vi "navX reading VI.vi"(0 "NavX Info In":T6, 1 "Mode":T7, 2 "error in (no error)":errorcluster) -> (3 "NavX Info Out":T6, 4 "NavX Readings":T4, 5 "Status":T3 {"OP Status" items=["INITIALIZING", "SELFTEST_IN_PROGRESS", "ERROR", "IMU_AUTOCAL_IN_PROGRESS", "NORMAL"]; "Calibration Status" items=["IMU_CAL_STATE_MASK"=3, "IMU_CAL_STATE_INPROGRESS"=0, "IMU_CAL_STATE_ACCUMULATE"=1, "IMU_CAL_STATE_COMPLETE"=2]}, 6 "Error Out":errorcluster)   [LabVIEW 2018]
uses:
  navX type def.ctl
  <vilib>/Studica/Studica Toolkit/Background/I2C Channel.ctl
  <vilib>/Studica/Studica Toolkit/NavX/TypeDefs/Flags/Z900_navX_Flags_OpStatusTypeDef.ctl
  <vilib>/Studica/Studica Toolkit/NavX/TypeDefs/Flags/Z900_navX_Flags_CalibrationStatusTypeDef.ctl
  <vilib>/Studica/Studica Toolkit/NavX/NavX.lvlib
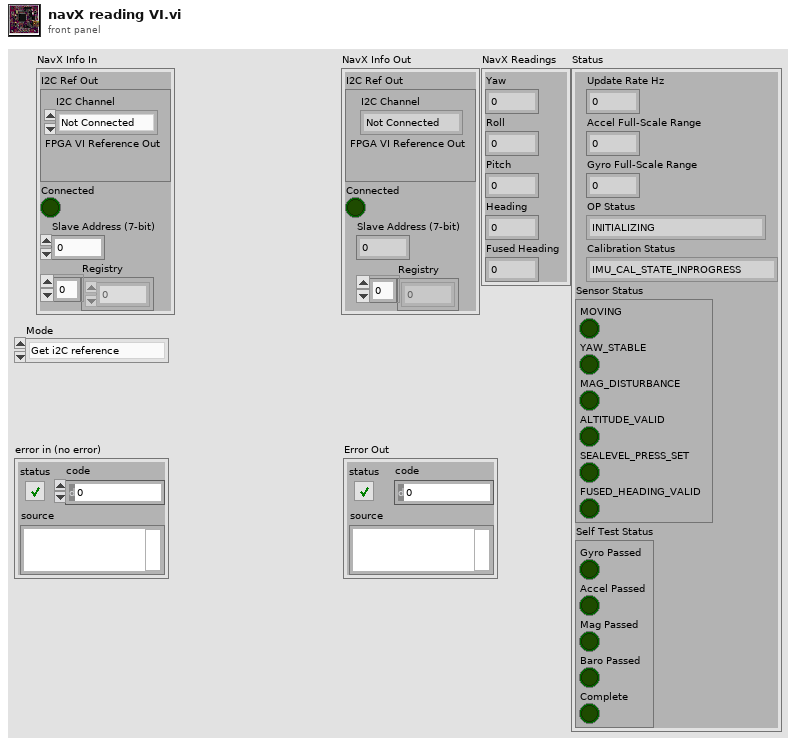
[diagram p1: front panel]
types:
  T1 = typedef "NavX.lvlib/Z900_navX_Flags_OpStatusTypeDef.ctl" = u8
  T2 = typedef "NavX.lvlib/Z900_navX_Flags_CalibrationStatusTypeDef.ctl" = u8
  T3 = cluster{"Update Rate Hz":u8, "Accel Full-Scale Range":u8, "Gyro Full-Scale Range":u16, "OP Status":T1, "Calibration Status":T2, "Sensor Status":cluster{"MOVING":bool, "YAW_STABLE":bool, "MAG_DISTURBANCE":bool, "ALTITUDE_VALID":bool, "SEALEVEL_PRESS_SET":bool, "FUSED_HEADING_VALID":bool}, "Self Test Status":cluster{"Gyro Passed":bool, "Accel Passed":bool, "Mag Passed":bool, "Baro Passed":bool, "Complete":bool}}
  T4 = cluster{"Yaw":dbl, "Roll":dbl, "Pitch":dbl, "Heading":dbl, "Fused Heading":dbl}
  T5 = typedef "I2C Channel.ctl" = enum16{"Not Connected", "A", "B"}
  T6 = cluster{"I2C Ref Out":cluster{"I2C Channel":T5, "FPGA VI Reference Out":refnum<k20>}, "Connected":bool, "Slave Address (7-bit)":u8, "Registry":u8[]}
  T7 = typedef "navX type def.ctl" = enum16{"Get i2C reference", "Read Values", "Zero Yaw"}
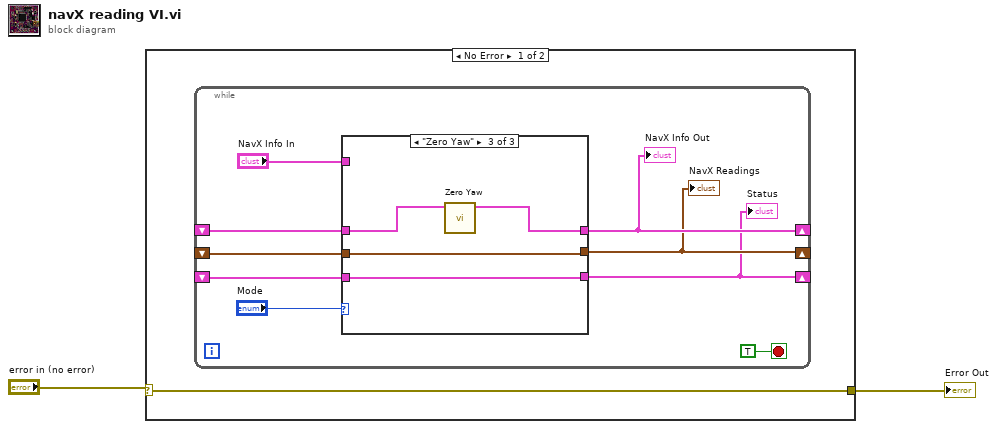
[diagram p0: block diagram]
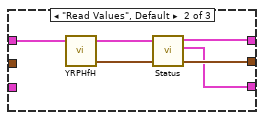
[diagram p3: hidden frame]
diagram:
  n1 = case shown="No Error" "error in (no error)" {
    selector: "error in (no error)" -> [w3 w25]
    tunnel: [w3 w25] -> w1
    frame No Error {
      n2 = while {
        shift-right: [w6] -> _
        shift-left: _ -> [w10]
        shift-right: [w5] -> _
        shift-left: _ -> [w9]
        shift-right: [w4] -> _
        shift-left: _ -> [w8]
        stop <- TRUE stop-if-true
        n3 = case shown="\"Zero Yaw\"" "Mode" {
          tunnel: "NavX Info In" -> [w15 _ _]
          tunnel: [w15 w18 w23] -> w6
          tunnel: w10 -> [_ w20 w24]
          tunnel: [w14 w17 w21] -> w5
          tunnel: [w13 w16 w22] -> w4
          tunnel: w9 -> [w14 _ w21]
          tunnel: w8 -> [w13 _ w22]
          frame "Get i2C reference" {
          }
          frame "Read Values", Default {
            n4 = call <vilib>:"YRPHfH.vi"("NavX Info In"=w20) -> ("YRPHfH"=w17:T4, "NavX Info Out"=w19:T6)  [unwired: 3 in]
            n5 = call <vilib>:"Status.vi"("NavX Info In"=w19) -> ("Status"=w16:T3, "NavX Info Out"=w18:T6)  [unwired: 9 in]
          }
          frame "Zero Yaw" {
            n6 = call <vilib>:"Zero Yaw.vi"("NavX Info In"=w24) -> ("NavX Info Out"=w23:T6)  [unwired: 10 in]
          }
        }
        "NavX Readings" <- w5
        "NavX Info Out" <- w6
        "Status" <- w4
      }
    }
    frame Error {
    }
  }
  "Error Out" <- w1
